vi "VI Scripting with Structures - Conditional Disable and Diagram Disable Structure.vi"   [LabVIEW 2019]
doc: "This example contains sample code demonstrating common VI Scripting navigational tasks relating to Conditional Disable Structures and Diagram Disable Structures."
panel:
  # "Overview: Illustrates several DisableStructure properties and methods used for inspecting and modifying Conditional Disable Structures and Diagram Disable Structures with VI Scripting.\nInstructions:\nOpen the block diagram of this VI to see several examples of properties and methods related to Disable Structures and VI Scripting.\n\nNote: Browse the diagram of this example to learn about VI Scripting concepts. This example is not meant to be run."
types:
  T1 = enum32{"Conditional Disable Style", "Diagram Disable Style"}
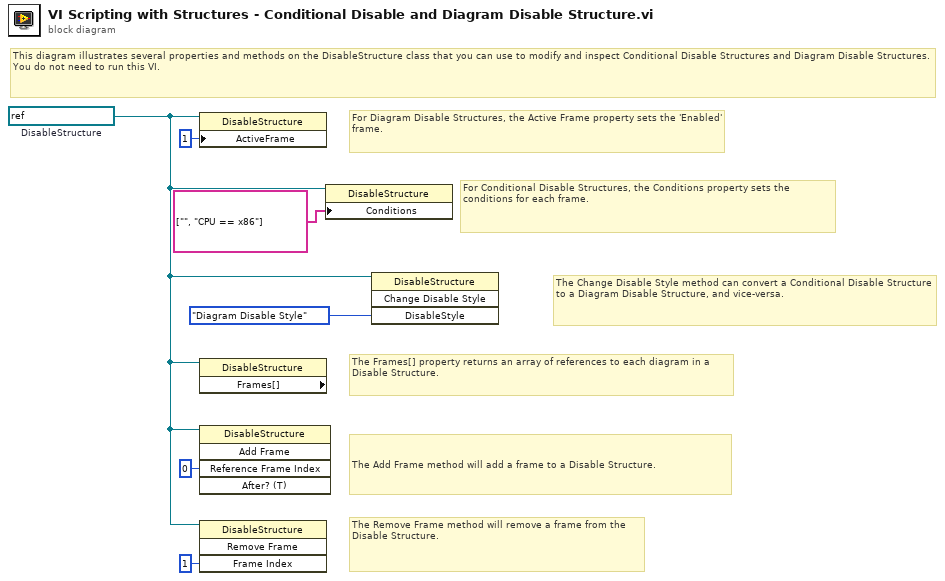
[diagram p0: block diagram]
diagram:
  w3 = refnum<vi> refnum  # DisableStructure
  # "The Remove Frame method will remove a frame from the Disable Structure."
  # "The Add Frame method will add a frame to a Disable Structure."
  # "The Frames[] property returns an array of references to each diagram in a Disable Structure."
  # "For Conditional Disable Structures, the Conditions property sets the conditions for each frame."
  # "This diagram illustrates several properties and methods on the DisableStructure class that you can use to modify and inspect Conditional Disable Structures and Diagram Disable Structures. You do not need to run this VI."
  # "The Change Disable Style method can convert a Conditional Disable Structure to a Diagram Disable Structure, and vice-versa."
  # "For Diagram Disable Structures, the Active Frame property sets the 'Enabled' frame."
  n1 = property class="DisableStructure"(reference=w3, "ActiveFrame"=i16 1 ("Active Frame")) -> ()  [unwired: 1 in, 2 out]
  n2 = property class="DisableStructure" props=["Frames[]"](reference=w3) -> ()  [unwired: 1 in, 3 out]
  n3 = invoke class="DisableStructure" method="Add Frame"(reference=w3, "Reference Frame Index"=u32 0) -> ()  [unwired: 3 in, 5 out]
  n4 = invoke class="DisableStructure" method="Remove Frame"(reference=w3, "Frame Index"=u32 1) -> ()  [unwired: 2 in, 4 out]
  n5 = property class="DisableStructure"(reference=w3, "Conditions"=string[] ["", "CPU == x86"]) -> ()  [unwired: 1 in, 2 out]
  n6 = invoke class="DisableStructure" method="Change Disable Style"(reference=w3, "DisableStyle"=T1."Diagram Disable Style" ("Disable Style")) -> ()  [unwired: 2 in, 4 out]
